vi "Get VIP Builder Config.vi"(8 "error in (no error)":errorcluster, 9 "Custom Parameters":string[](array[string]), 10 "Working Directory":path, 11 "Option Set in":refnum<class "Option Set.lvclass">) -> (0 "error out":errorcluster, 1 "Build Number Only":bool, 2 "New Version":string, 3 "VIPB Path":path, 4 "Set Version":bool, 5 "Output Directory":path, 7 "Copy To Output Dir":bool)   [LabVIEW 2011, in "G CLI VIP.lvlib"]
uses:
  G CLI VIP.lvlib
  <vilib>/Wiresmith Technology/G CLI/Argument Parser/Option Set Class/Option Set.lvclass
  <vilib>/Wiresmith Technology/G CLI/CLI Class/CLI.lvclass
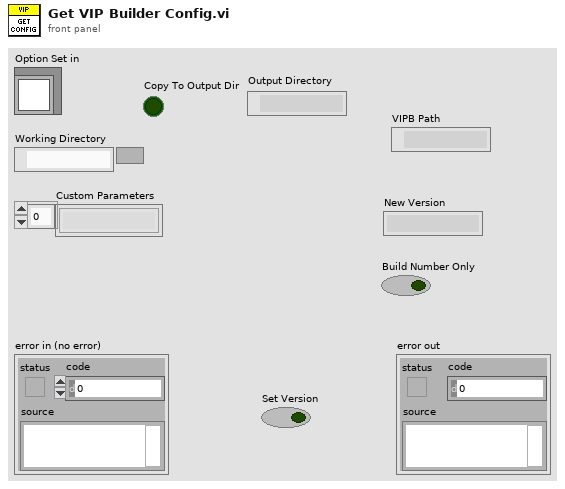
[diagram p1: front panel]
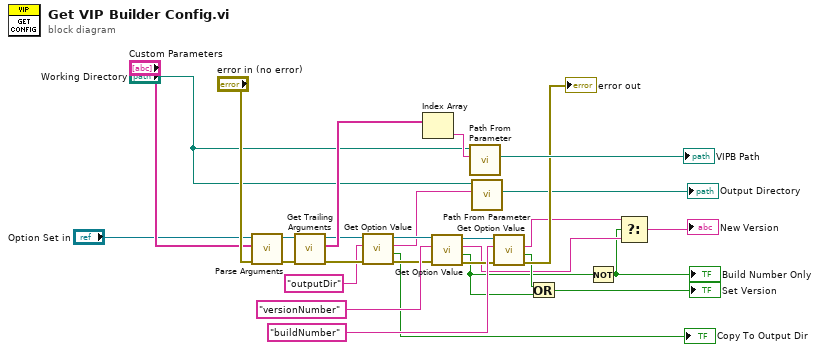
[diagram p0: block diagram]
diagram:
  n1 = call <vilib>:"Parse Arguments.vi"("error in (no error)"="error in (no error)", "Arguments"="Custom Parameters", "Option Set in"="Option Set in") -> ("error out"=w17:errorcluster, "Option Set out"=w18:refnum<class "Option Set.lvclass">)  [unwired: 5 in, 2 out]
  n2 = call <vilib>:"Get Trailing Arguments.vi"("error in (no error)"=w17, "Option Set in"=w18) -> ("error out"=w20:errorcluster, "Arguments"=w19:string[], "Option Set out"=w7:refnum<class "Option Set.lvclass">)  [unwired: 7 in]
  n3 = call <vilib>:"Get Option Value.vi"("error in (no error)"=w20, "Option Key"="outputDir", "Option Set in"=w7) -> ("error out"=w8:errorcluster, "Set"=→"Copy To Output Dir":bool, "Value"=w3:string, "Option Set out"=w6:refnum<class "Option Set.lvclass">)  [unwired: 5 in]
  n4 = Index Array(array=w19) -> (element=w14:string)  [unwired: 1 in]
  n5 = call <vilib>:"Get Option Value.vi"("error in (no error)"=w8, "Option Key"="versionNumber", "Option Set in"=w6) -> ("error out"=w23:errorcluster, "Set"=w11:bool, "Value"=w12:string, "Option Set out"=w24:refnum<class "Option Set.lvclass">)  [unwired: 5 in]
  n6 = call <vilib>:"Path From Parameter.vi"("Path Parameter"=w14, "Working Directory"="Working Directory") -> ("Full Path"=→"VIPB Path":path)  [unwired: 9 in]
  n7 = call <vilib>:"Path From Parameter.vi"("Path Parameter"=w3, "Working Directory"="Working Directory") -> ("Full Path"=→"Output Directory":path)  [unwired: 9 in]
  n8 = call <vilib>:"Get Option Value.vi"("error in (no error)"=w23, "Option Key"="buildNumber", "Option Set in"=w24) -> ("error out"=→"error out":errorcluster, "Set"=w26:bool, "Value"=w13:string)  [unwired: 5 in, 1 out]
  n9 = Or(x=w26, y=w11) -> (x .or. y?=→"Set Version":bool)
  n10 = Not(x=w11) -> (.not. x?=w9:bool)
  "Build Number Only" <- w9
  n11 = Select(t=w13, s=w9, f=w12) -> (s? t:f=→"New Version":string)
